vi "CRYPEAQ Partial Loudness.vi"(6 "Internal Noise":dbl[](array[numeric]), 8 "Nc":i32, 9 "fc":dbl[](array[numeric]), 10 "EPT":dbl[](array[numeric]), 11 "EPR":dbl[](array[numeric])) -> (3 "NL":dbl)   [LabVIEW 2013]
panel:
  out "XY Graph":cluster{"fc":dbl[], dbl[]}(graph)
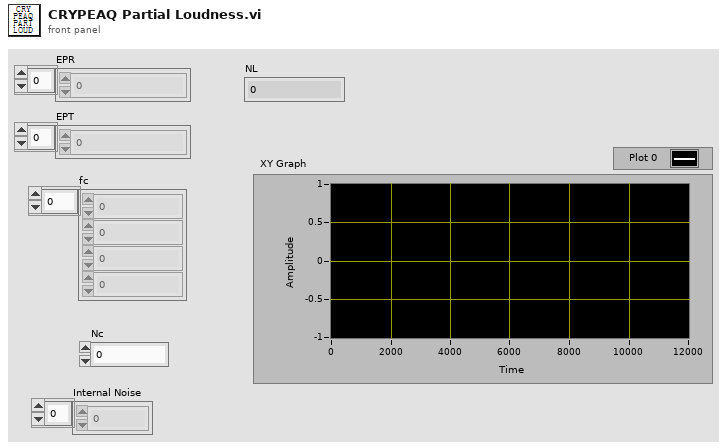
[diagram p1: front panel]
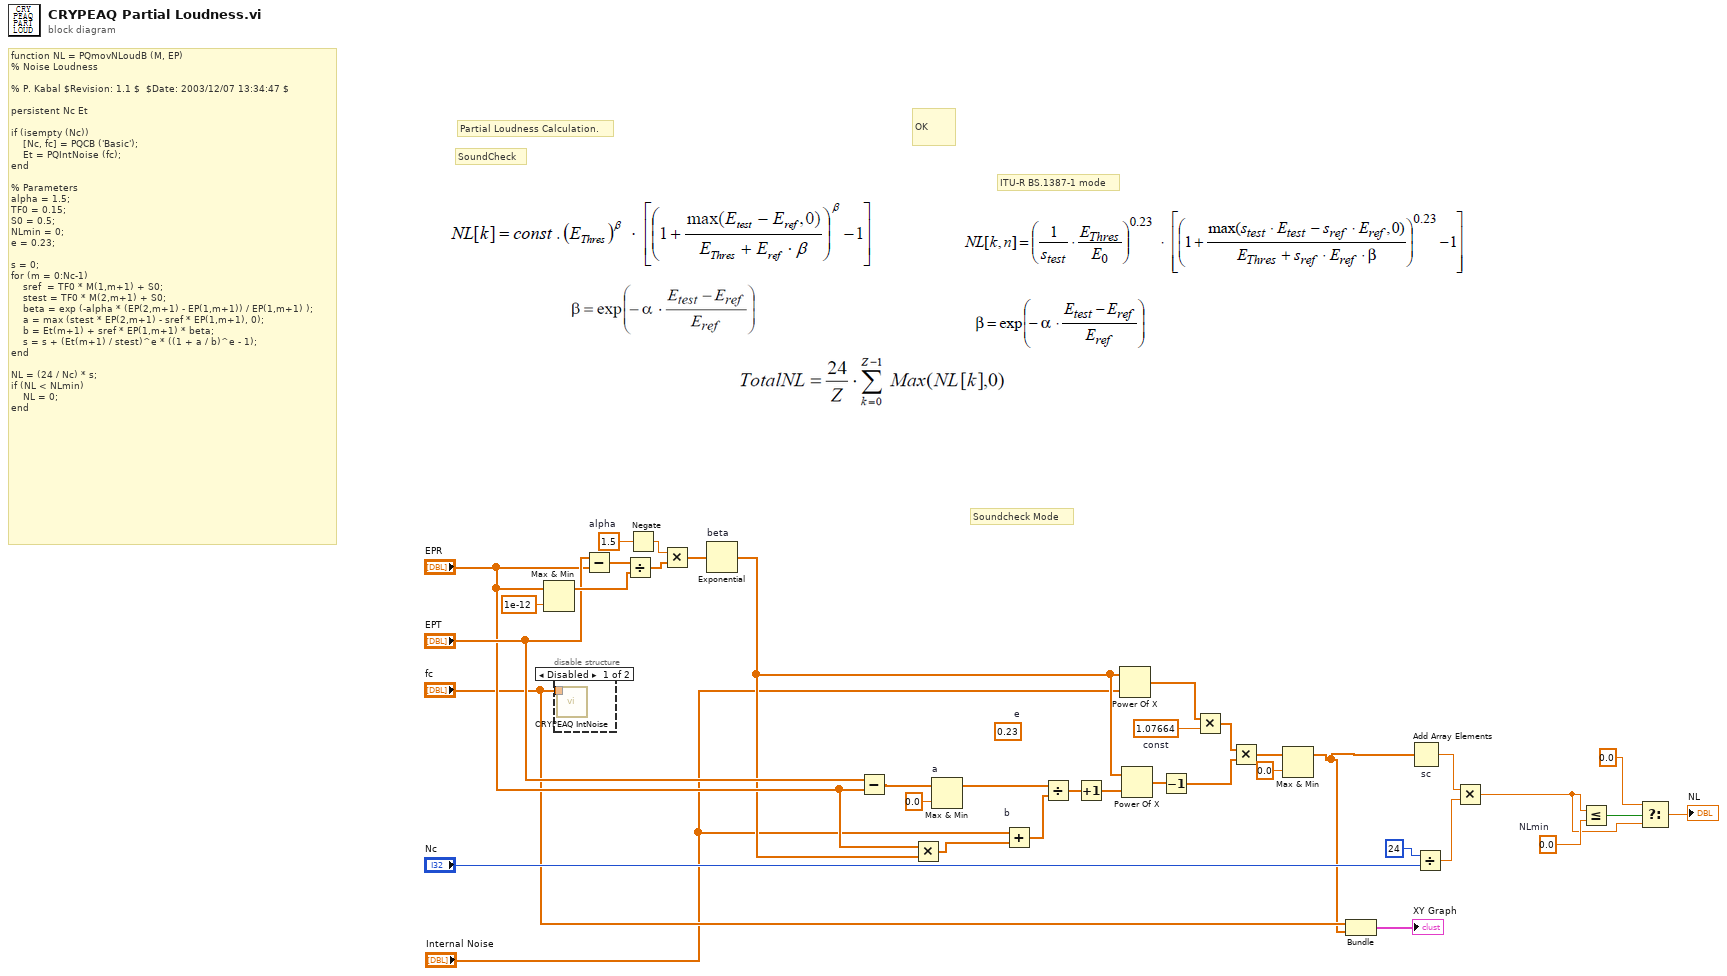
[diagram p0: block diagram]
diagram:
  w28 = 1.07664  # const
  w35 = 0.0  # NLmin
  w37 = 1.5  # alpha
  (unwired) 0.23  # e
  # "Soundcheck Mode"
  # "OK"
  # "ITU-R BS.1387-1 mode"
  # "SoundCheck"
  # "Partial Loudness Calculation."
  # "function NL = PQmovNLoudB (M, EP)\n% Noise Loudness\n\n% P. Kabal $Revision: 1.1 $  $Date: 2003/12/07 13:34:47 $\n\npersistent Nc Et\n\nif (isempty (Nc))\n    [Nc, fc] = PQCB ('Basic');\n    Et = PQIntNoise (fc);\nend\n\n% Parameters\nalpha = 1.5;\nTF0 = 0.15;\nS0 = 0.5;\nNLmin = 0;\ne = 0.23;\n\ns = 0;\nfor (m = 0:Nc-1)\n    sref  = TF0 * M(1,m+1) + S0;\n    stest = TF0 * M(2,m+1) + S0;\n    beta = exp (-alpha * (EP(2,m+1) - EP(1,m+1)) / EP(1,m+1) );\n    a = max (stest * EP(2,m+1) - sref * EP(1,m+1), 0);\n    b = Et(m+1) + sref * EP(1,m+1) * beta;\n    s = s + (Et(m+1) / stest)^e * ((1 + a / b)^e - 1);\nend\n\nNL = (24 / Nc) * s;\nif (NL < NLmin)\n    NL = 0;\nend"
  n1 = Max & Min(x="EPR", y=1e-12) -> (max(x,y)=w14:dbl[])  [unwired: 1 out]
  n2 = disable-structure shown="Disabled" {
    disable-tunnel: "fc" -> [w38 _]
    frame Disabled {
      n3 = call "CRYPEAQ IntNoise.vi"("fc"=w38) -> ()  [unwired: 10 in, 1 out]
    }
    frame Enabled {
    }
  }
  n4 = Subtract(x="EPT", y="EPR") -> (x-y=w30:dbl[])
  n5 = Divide(x=w30, y=w14) -> (x/y=w29:dbl[])
  n6 = Negate(x=w37) -> (-x=w31:dbl)
  n7 = Multiply(x=w31, y=w29) -> (x*y=w16:dbl[])
  n8 = Exponential "beta"(1:w16) -> (0:w3:dbl[])
  n9 = Subtract(x="EPT", y="EPR") -> (x-y=w25:dbl[])
  n10 = Multiply(x="EPR", y=w3) -> (x*y=w23:dbl[])
  n11 = Max & Min "a"(x=w25, y=0.0) -> (max(x,y)=w24:dbl[])  [unwired: 1 out]
  n12 = Add "b"(x="Internal Noise", y=w23) -> (x+y=w22:dbl[])
  n13 = Divide(x=w24, y=w22) -> (x/y=w21:dbl[])
  n14 = Increment(x=w21) -> (x+1=w19:dbl[])
  n15 = Power Of X(1:"Internal Noise", 2:w3) -> (0:w27:dbl[])
  n16 = Power Of X(1:w19, 2:w3) -> (0:w20:dbl[])
  n17 = Decrement(x=w20) -> (x-1=w17:dbl[])
  n18 = Multiply(x=w27, y=w28) -> (x*y=w18:dbl[])
  n19 = Multiply(x=w18, y=w17) -> (x*y=w10:dbl[])
  n20 = Max & Min(x=w10, y=0.0) -> (max(x,y)=w1:dbl[])  [unwired: 1 out]
  n21 = Bundle("fc"="fc", w1) -> (→"XY Graph":cluster{"fc":dbl[], dbl[]})  [unwired: 1 in]
  n22 = Add Array Elements "sc"(numeric array=w1) -> (sum=w7:dbl)
  n23 = Divide(x=24, y="Nc") -> (x/y=w36:dbl)
  n24 = Multiply(x=w7, y=w36) -> (x*y=w5:dbl)
  n25 = Less Or Equal?(x=w5, y=w35) -> (x <= y?=w34:bool)
  n26 = Select(t=0.0, s=w34, f=w5) -> (s? t:f=→"NL":dbl)
